vi "冗余度编码.vi"() -> ()   [LabVIEW 2020]
panel:
  out "输出编码：":string
  out "T":dbl
  out "Array":dbl[](array[numeric])
  in  "Q":dbl=2.0
  out "N":i32
  in  "输入序列":bool[](array[boolean])=[FALSE, FALSE, TRUE, FALSE, FALSE, FALSE, FALSE, FALSE, FALSE, FALSE, TRUE, FALSE, FALSE, FALSE, FALSE]
  # "冗余度编码"
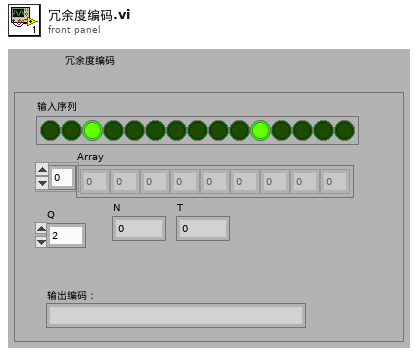
[diagram p1: front panel]
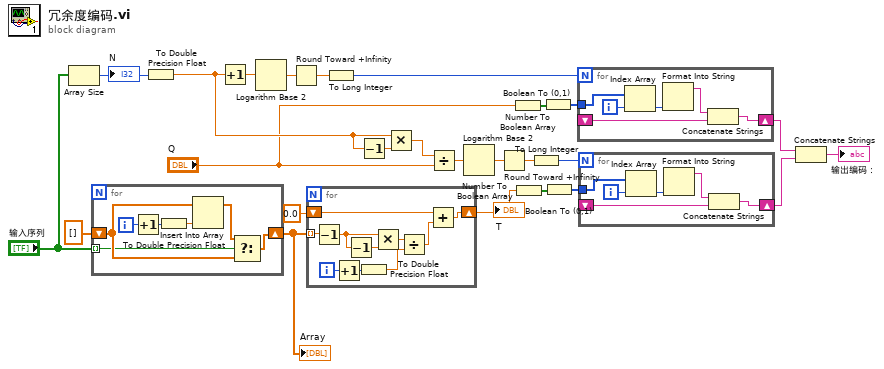
[diagram p0: block diagram]
diagram:
  n1 = Array Size(array="输入序列") -> (size(s)=w17:i32)
  "N" <- w17
  n2 = for {
    tunnel: "输入序列" -> [w28] mode=indexing
    shift-right: [w29] -> w23
    shift-left: dbl[] [] -> [w30]
    i -> [w32]
    n3 = Increment(x=w32) -> (x+1=w27:i32)
    n4 = To Double Precision Float(number=w27) -> (double precision float=w26:dbl)
    n5 = Insert Into Array(array=w30, new element=w26) -> (w31:dbl[])  [unwired: 1 in]
    n6 = Select(t=w31, s=w28, f=w30) -> (s? t:f=w29:dbl[])
  }
  "Array" <- w23
  n7 = To Double Precision Float(number=w17) -> (double precision float=w16:dbl)
  n8 = Increment(x=w16) -> (x+1=w21:dbl)
  n9 = Logarithm Base 2(1:w21) -> (0:w20:dbl)
  n10 = Round Toward +Infinity(x=w20) -> (ceil(x): smallest int >= x=w13:dbl)
  n11 = for {
    tunnel: w23 -> [w41] mode=indexing
    shift-right: [w33] -> w5
    shift-left: 0.0 -> [w35]
    i -> [w39]
    n12 = Decrement(x=w41) -> (x-1=w40:dbl)
    n13 = Increment(x=w39) -> (x+1=w37:i32)
    n14 = Decrement(x=w40) -> (x-1=w42:dbl)
    n15 = To Double Precision Float(number=w37) -> (double precision float=w36:dbl)
    n16 = Multiply(x=w40, y=w42) -> (x*y=w38:dbl)
    n17 = Divide(x=w38, y=w36) -> (x/y=w34:dbl)
    n18 = Add(x=w35, y=w34) -> (x+y=w33:dbl)
  }
  "T" <- w5
  n19 = To Long Integer(number=w13) -> (32bit integer=w8:i32)
  n20 = Decrement(x=w16) -> (x-1=w18:dbl)
  n21 = Multiply(x=w16, y=w18) -> (x*y=w19:dbl)
  n22 = Divide(x=w19, y="Q") -> (x/y=w14:dbl)
  n23 = Logarithm Base 2(1:w14) -> (0:w15:dbl)
  n24 = Round Toward +Infinity(x=w15) -> (ceil(x): smallest int >= x=w12:dbl)
  n25 = Number To Boolean Array(number="Q") -> (Boolean array=w11:bool[])
  n26 = Number To Boolean Array(number=w5) -> (Boolean array=w6:bool[])
  n27 = To Long Integer(number=w12) -> (32bit integer=w1:i32)
  n28 = Boolean To (0,1)(Boolean=w11) -> (0, 1=w10:i16[])
  n29 = Boolean To (0,1)(Boolean=w6) -> (0, 1=w7:i16[])
  n30 = for {
    N: w8 -> [_]
    tunnel: w10 -> [w45]
    shift-right: [w48] -> w4
    shift-left: _ -> [w46]
    i -> [w44]
    n31 = Index Array(array=w45, index=w44) -> (element=w43:i16)
    n32 = Format Into String(w43) -> (resulting string=w47:string)  [unwired: 3 in, 1 out]
    n33 = Concatenate Strings(w47, w46) -> (w48:string)
  }
  n34 = for {
    N: w1 -> [_]
    tunnel: w7 -> [w51]
    shift-right: [w54] -> w3
    shift-left: _ -> [w52]
    i -> [w50]
    n35 = Index Array(array=w51, index=w50) -> (element=w49:i16)
    n36 = Format Into String(w49) -> (resulting string=w53:string)  [unwired: 3 in, 1 out]
    n37 = Concatenate Strings(w53, w52) -> (w54:string)
  }
  n38 = Concatenate Strings(w4, w3) -> (→"输出编码：":string)
